vi "Output Drive.vi"(8 "error in (no error)":errorcluster, 11 "TeleOp Data Cluster":T1) -> (0 "error out":errorcluster)   [LabVIEW 2018]
uses:
  TypeDefs/Teleop Data Cluster.ctl
  TypeDefs/Joystick Buttons.ctl
  TypeDefs/typedef_enum_Refnums.ctl
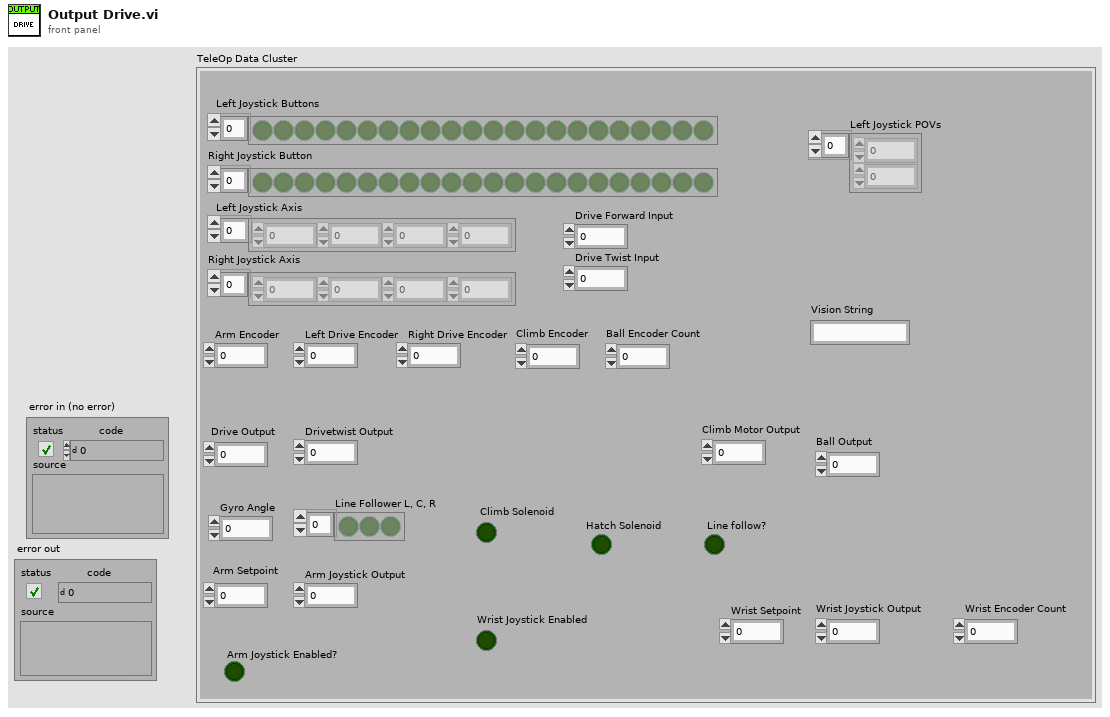
[diagram p1: front panel]
types:
  T1 = typedef "Teleop Data Cluster.ctl" = cluster{"Drive Forward Input ":dbl, "Drive Twist Input":dbl, "Drive Output":dbl, "Drivetwist Output":dbl, "Left Joystick Buttons":bool[], "Left Joystick Axis":dbl[], "Right Joystick Axis":dbl[], "Right Joystick Button":bool[], "Arm Encoder":dbl, "Left Drive Encoder":dbl, "Right Drive Encoder":dbl, "Gyro Angle ":dbl, "Arm Joystick Output  ":dbl, "Line Follower L, C, R ":bool[], "Line follow?":bool, " Climb Solenoid":bool, "Wrist Encoder Count":dbl, "Wrist Joystick Output":dbl, "Ball Encoder Count":dbl, "Ball Output":dbl, "Climb Encoder":dbl, "Climb Motor Output":dbl, " Hatch Solenoid":bool, "Arm Setpoint ":dbl, "Wrist Setpoint ":dbl, "Arm Joystick Enabled?":bool, "Wrist Joystick Enabled":bool, "Vision String":string, "Left Joystick POVs":i16[]}
  T2 = typedef "Joystick Buttons.ctl" = enum16{"Trigger", "Thumb", "Top 3", "Top 4", "Top 5", "Top 6", "Bottom 7", "Bottom 8", "Bottom 9", "Bottom 10", "Bottom 11", "Bottom 12"}
  T3 = typedef "typedef_enum_Refnums.ctl" = enum16{"Ball_Encoder", "Ball_Motor", "Camera", "Linefollow_3", "Linefollow_2", "Linefollow_1", "Gyro", "Hatch_Solenoid", "Climb_Back_Solenoid", "Arm_Encoder", "Arm_Motor", "Lift_Encoder", "Drive", "Drive_Motor_R", "Drive_Motor_L", "Drive_Encoder_R", "Drive_Encoder_L", "Joy_R", "Joy_L", "Wrist_Motor", "Wrist_Encoder", "Climb Upper Limit", "Climb Lower Limit ", "Climb_Front_Motor"}
  T4 = typedef "CTRE_PigeonIMU_DeviceRef.ctl" = cluster{"DeviceStatus":errorcluster, "Device Number":u8, "Type":T5, "Device ID":u32, "Handle":u64, "UsageFrame":u32, "Library Path":path}
  T5 = typedef "CTRE_PigeonIMU_ConnectionType.ctl" = u32
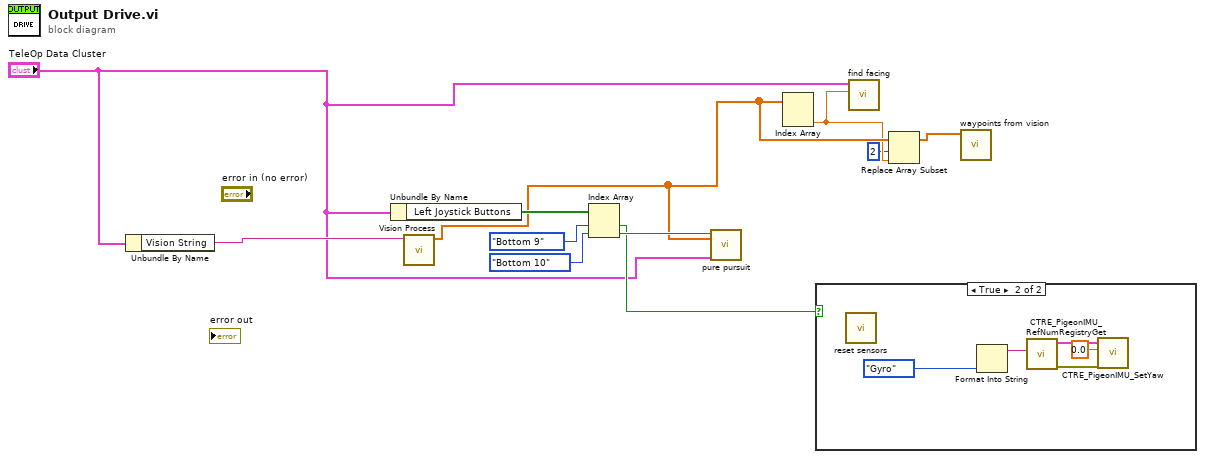
[diagram p0: block diagram]
diagram:
  n1 = Unbundle By Name("TeleOp Data Cluster") -> ("Vision String"=w6:string)
  n2 = Unbundle By Name("TeleOp Data Cluster") -> ("Left Joystick Buttons"=w11:bool[])
  n3 = call "Vision Process.vi"("Vision String"=w6) -> ("Default Values"=w4:dbl[])  [unwired: 10 in]
  n4 = Index Array(array=w11, index #1=Joystick_Buttons."Bottom 9" ("Enum"), index #2=Joystick_Buttons."Bottom 10" ("Enum")) -> (element #1=w7:bool, element #2=w8:bool)
  n5 = call "pure pursuit.vi"("input cluster"="TeleOp Data Cluster", "Vision Data"=w4, "Button"=w8) -> ()  [unwired: 9 in]
  n6 = Index Array(array=w4) -> (element #2=w3:dbl)  [unwired: 2 in, 1 out]
  n7 = case shown="True" w7 {
    frame False {
    }
    frame True {
      n8 = call "reset sensors.vi"() -> ()  [unwired: 12 in]
      n9 = Format Into String(typedef_enum_Refnums."Gyro" ("RefNums")) -> (resulting string=w12:string)  [unwired: 3 in, 1 out]
      n10 = call <vilib>:"CTRE_PigeonIMU_RefNumRegistryGet.vi"("refnum name"=w12) -> ("error out"=w16:errorcluster, "PigeonIMUDevRef"=w15:T4)  [unwired: 9 in]
      n11 = call <vilib>:"CTRE_PigeonIMU_SetYaw.vi"("error in (no error)"=w16, "Value"=0.0, "PigeonIMUDevRef"=w15) -> ()  [unwired: 7 in, 2 out]
    }
  }
  n12 = call "find facing.vi"("Robot Angle"=w3, "TeleOp Data Cluster"="TeleOp Data Cluster") -> ()  [unwired: 9 in, 1 out]
  n13 = Replace Array Subset(array=w4, new element=w3, index=2) -> (w1:dbl[])
  n14 = call "waypoints from vision.vi"("Vision Data"=w1) -> ()  [unwired: 10 in, 1 out]
